vi "Pass-Messages.vi"(8 "error in":errorcluster, 11 "Message":T1) -> (0 "error out":errorcluster, 1 "Value":string, 2 "Source":string, 3 "Name":string)   [LabVIEW 2016]
uses:
  RT-Typedefinitions/RT-Message-Type.ctl
  <vilib>/NI/STM/TCP/Write Message (TCP).vi
  <vilib>/NI/STM/NI STM.lvlib
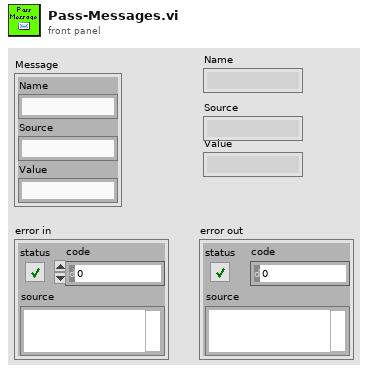
[diagram p1: front panel]
types:
  T1 = typedef "RT-Message-Type.ctl" = cluster{"Name":string, "Source":string, "Value":string}
  T2 = enum16{"Read", "Delete", "SetElement", "GetElement", "GetFPelements"}
  T3 = typedef "NI STM.lvlib/TCP Connection Info.ctl" = cluster{"connection ID":refnum<k5>, "meta data":T4[]}
  T4 = typedef "NI STM.lvlib/MetaDataElement.ctl" = string
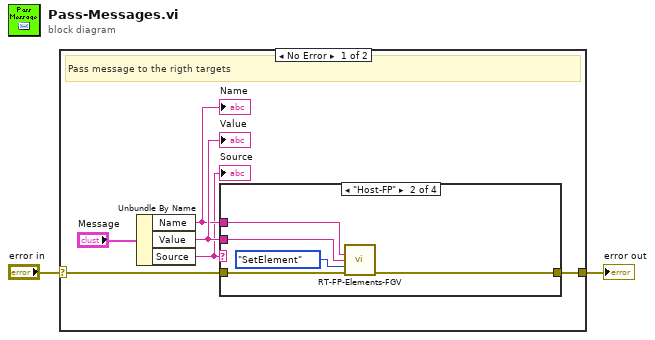
[diagram p0: block diagram]
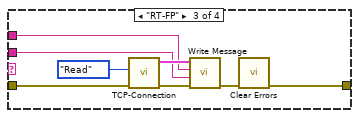
[diagram p3: hidden frame]
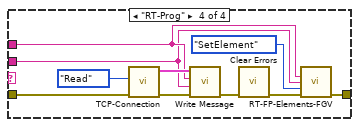
[diagram p4: hidden frame]
diagram:
  n1 = case shown="No Error" "error in" {
    selector: "error in" -> [w6 w33]
    tunnel: [w7 w33] -> w2
    frame No Error {
      # "Pass message to the rigth targets"
      n2 = Unbundle By Name("Message") -> ("Name"=w4:string, "Value"=w5:string, "Source"=w3:string)
      "Name" <- w4
      "Value" <- w5
      "Source" <- w3
      n3 = case shown="\"Host-FP\"" w3 {
        tunnel: w6 -> [w9 w14 w22 w32]
        tunnel: [w9 w13 w15 w26] -> w7
        tunnel: w4 -> [_ w12 w16 w24]
        tunnel: w5 -> [_ w11 w17 w23]
        frame "False", Default {
        }
        frame "Host-FP" {
          n4 = call "RT-FP-Elements-FGV.vi"("Name"=w12, "Value in"=w11, "Mode"=T2."SetElement", "error in"=w14) -> ("error out"=w13:errorcluster)  [unwired: 7 in, 4 out]
        }
        frame "RT-FP" {
          n5 = call "TCP-Connection.vi"("error in"=w22, "Mode"=enum16{"TCP-Lost", "Write", "Read"}."Read") -> ("error out"=w19:errorcluster, "connection info Out"=w18:T3)  [unwired: 7 in, 1 out]
          n6 = call-poly <vilib>:"Write Message.vi"("error in"=w19, "data"=w17, "name"=w16, "connection info in"=w18) -> ("error out"=w20:errorcluster)  [unwired: 6 in, 1 out]
          n7 = call <vilib>:"Clear Errors.vi"("error in (no error)"=w20) -> ("error out"=w15:errorcluster)  [unwired: 5 in, 1 out]
        }
        frame "RT-Prog" {
          n8 = call "TCP-Connection.vi"("error in"=w32, "Mode"=enum16{"TCP-Lost", "Write", "Read"}."Read") -> ("error out"=w29:errorcluster, "connection info Out"=w28:T3)  [unwired: 7 in, 1 out]
          n9 = call-poly <vilib>:"Write Message.vi"("error in"=w29, "data"=w23, "name"=w24, "connection info in"=w28) -> ("error out"=w30:errorcluster)  [unwired: 6 in, 1 out]
          n10 = call <vilib>:"Clear Errors.vi"("error in (no error)"=w30) -> ("error out"=w27:errorcluster)  [unwired: 5 in, 1 out]
          n11 = call "RT-FP-Elements-FGV.vi"("Name"=w24, "Value in"=w23, "Mode"=T2."SetElement", "error in"=w27) -> ("error out"=w26:errorcluster)  [unwired: 7 in, 4 out]
        }
      }
    }
    frame Error {
    }
  }
  "error out" <- w2
